vi "Swap_DBL.vi"(4 "Swap(T)":bool=TRUE, 6 "b":dbl=1.0, 7 "a":dbl=1.0) -> (1 "b":dbl=1.0 format="%.2f", 2 "a":dbl=1.0 format="%.2f")   [LabVIEW 2012]
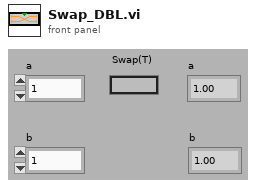
[diagram p1: front panel]
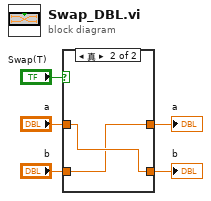
[diagram p0: block diagram]
diagram:
  n1 = case shown="真" "Swap(T)" {
    tunnel: "a" -> [w7 w9]
    tunnel: "b" -> [w6 w8]
    tunnel: [w7 w8] -> w2
    tunnel: [w6 w9] -> w1
    frame False {
    }
    frame True {
    }
  }
  "a" <- w2
  "b" <- w1
